vi "showBG.vi"() -> ()   [LabVIEW 2020]
panel:
  out "Ch4 BG":dbl[](graph)
  in  "OK Button":bool
  out "Ch3 BG":dbl[](graph)
  out "Ch2 BG":dbl[](graph)
  out "Ch1 BG":dbl[](graph)
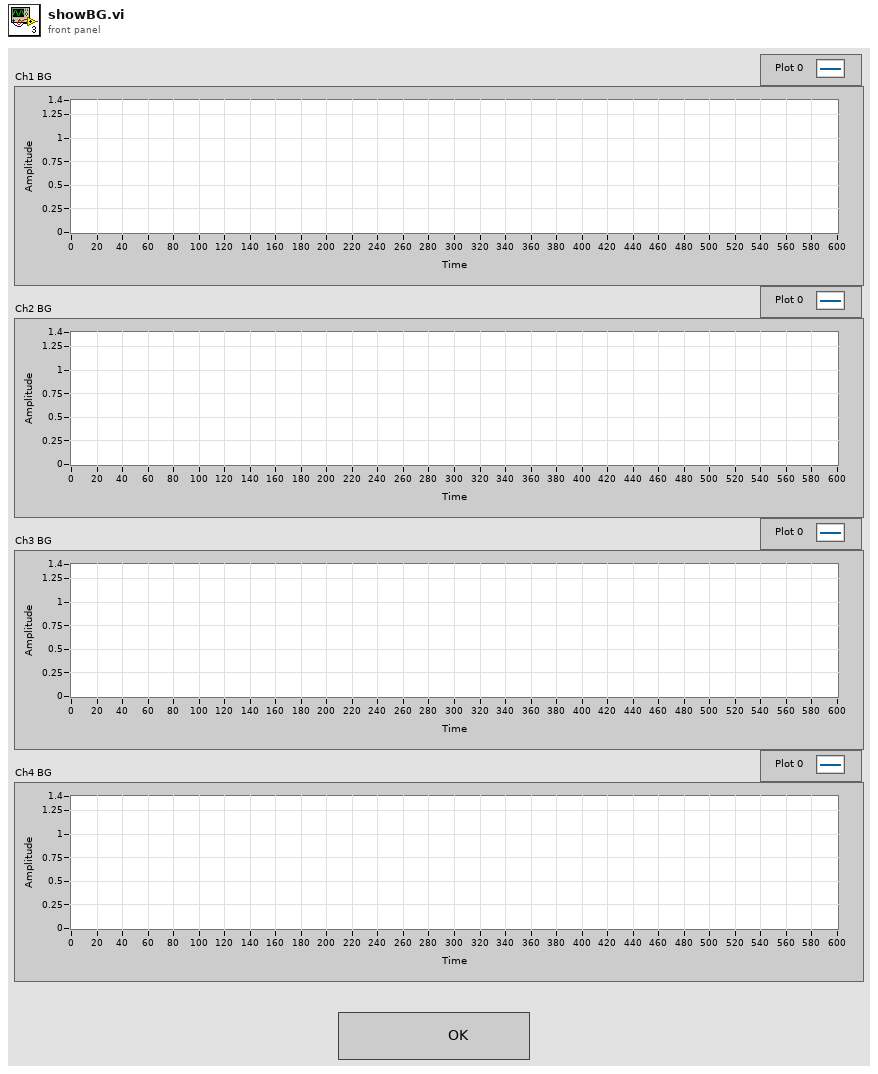
[diagram p1: front panel]
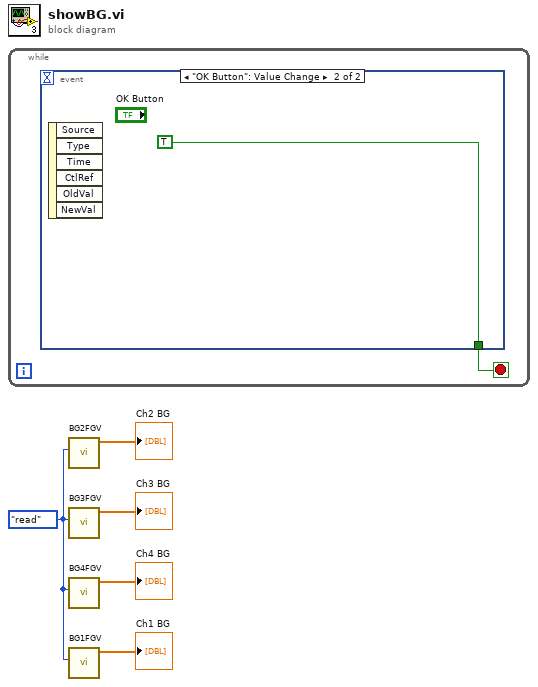
[diagram p0: block diagram]
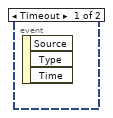
[diagram p2: hidden frame]
diagram:
  w2 = enum16{"write", "read"}."read" ("action")
  n1 = while {
    stop <- w6 stop-if-true
    n2 = event shown="[1] \"OK Button\": Value Change" {
      selector: _ -> [_ _]
      dyn-events: _ -> [_ _]
      timeout: _ -> [_ _]
      tunnel: [_ TRUE] -> w6
      event Timeout {
        n3 = event-data() -> ()  [unwired: 1 in, 3 out]
      }
      event "OK Button": Value Change {
        n4 = event-data() -> ()  [unwired: 1 in, 6 out]
      }
    }
  }
  n5 = call "BG2FGV.vi"("action"=w2) -> ("BG2 out"=→"Ch2 BG":dbl[])  [unwired: 9 in, 1 out]
  n6 = call "BG3FGV.vi"("action"=w2) -> ("BG3 out"=→"Ch3 BG":dbl[])  [unwired: 9 in, 1 out]
  n7 = call "BG4FGV.vi"("action"=w2) -> ("BG14out"=→"Ch4 BG":dbl[])  [unwired: 9 in, 1 out]
  n8 = call "BG1FGV.vi"("action"=w2) -> ("BG1 out"=→"Ch1 BG":dbl[])  [unwired: 9 in, 1 out]
